vi "DAC Configure FP View.vi"(8 "error in":errorcluster, 11 "DAC HS Vib in":refnum<class "DAC HS Vib.lvclass">) -> (0 "error out":errorcluster, 3 "DAC HS Vib out":refnum<class "DAC HS Vib.lvclass">)   [LabVIEW 2019, in "DAC.lvlib" / "DAC HS Vib.lvclass"]
uses:
  DAC HS Vib.lvclass
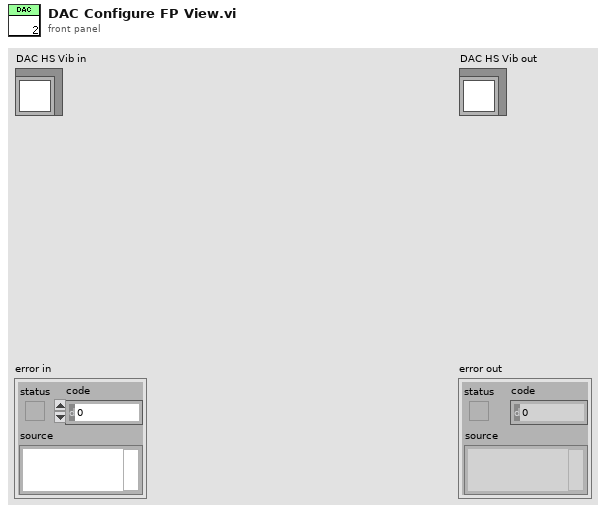
[diagram p1: front panel]
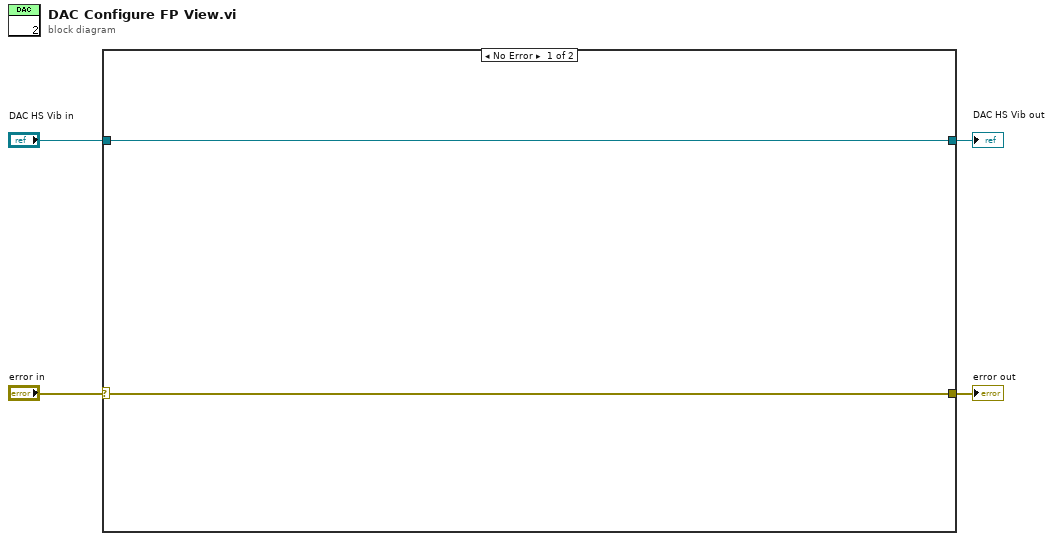
[diagram p0: block diagram]
diagram:
  n1 = case shown="No Error" "error in" {
    selector: "error in" -> [w5 w8]
    tunnel: [w5 w8] -> w1
    tunnel: [w6 w7] -> w2
    tunnel: "DAC HS Vib in" -> [w6 w7]
    frame No Error {
    }
    frame Error {
    }
  }
  "error out" <- w1
  "DAC HS Vib out" <- w2
